vi "HTTP.Get Header.vi"(8 "error in (no error)":errorcluster, 10 "Header Name":T1, 11 "Connection.WS in":refnum<class "Connection.WS.lvclass">) -> (0 "error out":errorcluster, 1 "found":bool, 2 "Value":string, 3 "Connection.WS out":refnum<class "Connection.WS.lvclass">)   [LabVIEW 2013, in "Connection.WS_GOSPL.lvlib" / "Connection.WS.lvclass"]
uses:
  Connection.WS.lvclass
  Header Fields -- combo.ctl
  Connection.WS.lvclass/Connection.WS.ctl
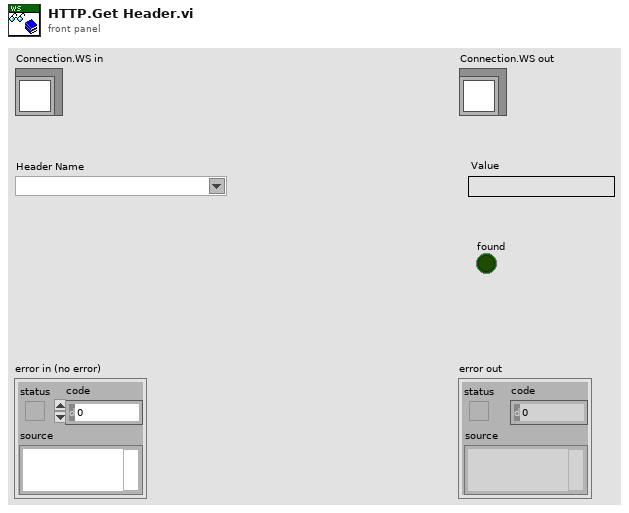
[diagram p1: front panel]
types:
  T1 = typedef "Connection.WS_GOSPL.lvlib/Connection.WS.lvclass/Header Fields -- combo.ctl" = string
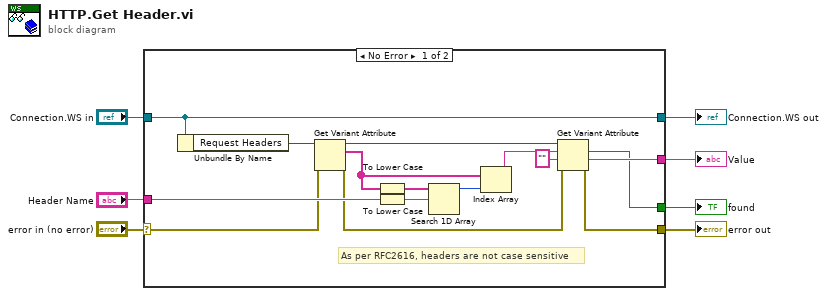
[diagram p0: block diagram]
diagram:
  n1 = case shown="No Error" "error in (no error)" {
    selector: "error in (no error)" -> [w9 w24]
    tunnel: [w10 w24] -> w6
    tunnel: [w22 w23] -> w4
    tunnel: "Connection.WS in" -> [w22 w23]
    tunnel: "Header Name" -> [w19 _]
    tunnel: [w13 _] -> w2
    tunnel: [w12 _] -> w1
    frame No Error {
      # "As per RFC2616, headers are not case sensitive"
      n2 = Unbundle By Name(w22) -> ("Request Headers"=w21:variant)
      n3 = Get Variant Attribute(Variant=w21, error in=w9) -> (duplicate Variant=w16:variant, names=w17:string[], error out=w8:errorcluster)  [unwired: 2 in, 1 out]
      n4 = To Lower Case(string=w17) -> (all lower case string=w20:string[])
      n5 = To Lower Case(string=w19) -> (all lower case string=w18:T1)
      n6 = Search 1D Array(1D array=w20, element=w18) -> (index of element=w11:i32)  [unwired: 1 in]
      n7 = Index Array(array=w17, index=w11) -> (element=w15:string)
      n8 = Get Variant Attribute(Variant=w16, name=w15, default value (empty Variant)="", error in=w8) -> (found=w12:bool, value=w13:string, error out=w10:errorcluster)  [unwired: 1 out]
    }
    frame Error {
    }
  }
  "error out" <- w6
  "Connection.WS out" <- w4
  "Value" <- w2
  "found" <- w1
